vi "Get Triggered Block.vi"(8 "error in (no error)":errorcluster, 9 "Post-trigger points":i32, 10 "Pre-trigger points":i32, 11 "RP Instrument in":refnum<class "RP Instrument.lvclass">) -> (0 "error out":errorcluster, 2 "Data out":string, 3 "RP Instrument out":refnum<class "RP Instrument.lvclass">)   [LabVIEW 2024, in "RP Instrument.lvclass"]
uses:
  RP Instrument.lvclass
  RP Instrument.lvclass/RP Instrument.ctl
  Read Samples per trigger increment .vi
  Read Bytes per sample.vi
  RP Communicator/RP Communicator.lvclass
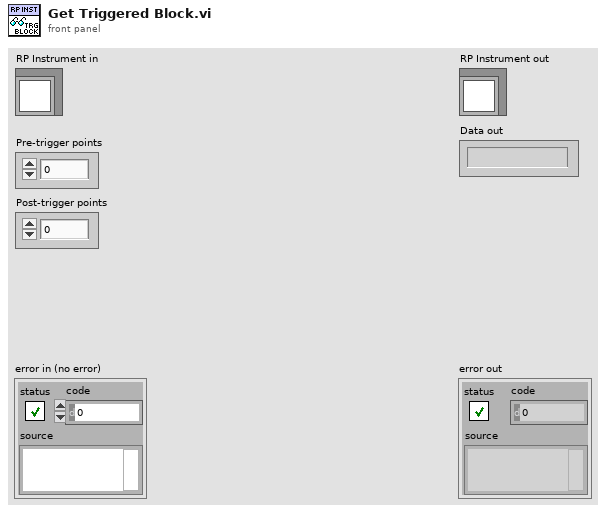
[diagram p1: front panel]
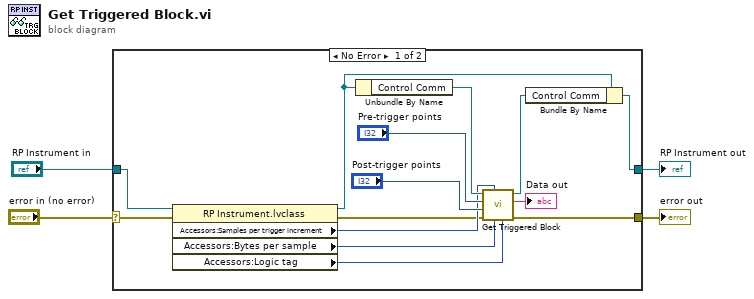
[diagram p0: block diagram]
diagram:
  n1 = case shown="No Error" "error in (no error)" {
    selector: "error in (no error)" -> [w6 w20]
    tunnel: [w13 w20] -> w3
    tunnel: [w15 w19] -> w1
    tunnel: "RP Instrument in" -> [w16 w19]
    frame No Error {
      n2 = property class="RP Instrument.lvclass"(reference=w16, error in=w6) -> (reference out=w10:refnum<class "RP Instrument.lvclass">, error out=w5:errorcluster, "Accessors:Samples per trigger increment "=w8:i32, "Accessors:Bytes per sample"=w7:i32, "Accessors:Logic tag"=w9:u16)
      n3 = Unbundle By Name(w10) -> ("Control Comm"=w18:refnum<class "RP Communicator.lvclass">)
      n4 = call-dynamic "Get Triggered Block.vi"("Logic tag"=w9, "Bytes per sample"=w7, "Samples per trigger increment"=w8, "error in (no error)"=w5, "Post-trigger samples"="Post-trigger points", "Pre-trigger samples"="Pre-trigger points", "RP Communicator in"=w18) -> ("error out"=w13:errorcluster, "data out"=→"Data out":string, "RP Communicator out"=w17:refnum<class "RP Communicator.lvclass">)  [unwired: 2 in]
      n5 = Bundle By Name(cluster=w10, "Control Comm"=w17) -> (w15:refnum<class "RP Instrument.lvclass">)
    }
    frame Error {
    }
  }
  "error out" <- w3
  "RP Instrument out" <- w1
